vi "Turn To X -no loop.vi"(3 "STOP?":bool, 4 "Dest":u16, 5 "Start":u16, 6 "error in":errorcluster, 7 "FPGA VI Reference in":refnum<k20>) -> (0 "error out":errorcluster, 1 "FPGA VI Reference Out":refnum<k20>, 2 "x-y":i16)   [LabVIEW 2014]
uses:
  <vilib>/Utility/error.llb/Error Cluster From Error Code.vi
  <vilib>/rvi/errors/niLvFpgaAdjustHostInterfaceError.vi
  <vilib>/rvi/interface/nirviReadWriteControl/nirviReadWriteControl.xnode
  NiFpgaLv.dll
  <vilib>/rvi/interface/Simulation/niFpgaSimulationCallBeginRW.vi
panel:
  out "16bit integer":i16
  in  "Friction":dbl=1.0
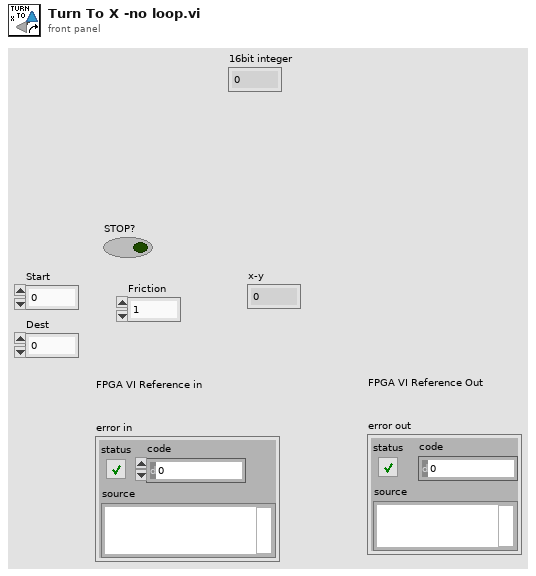
[diagram p1: front panel]
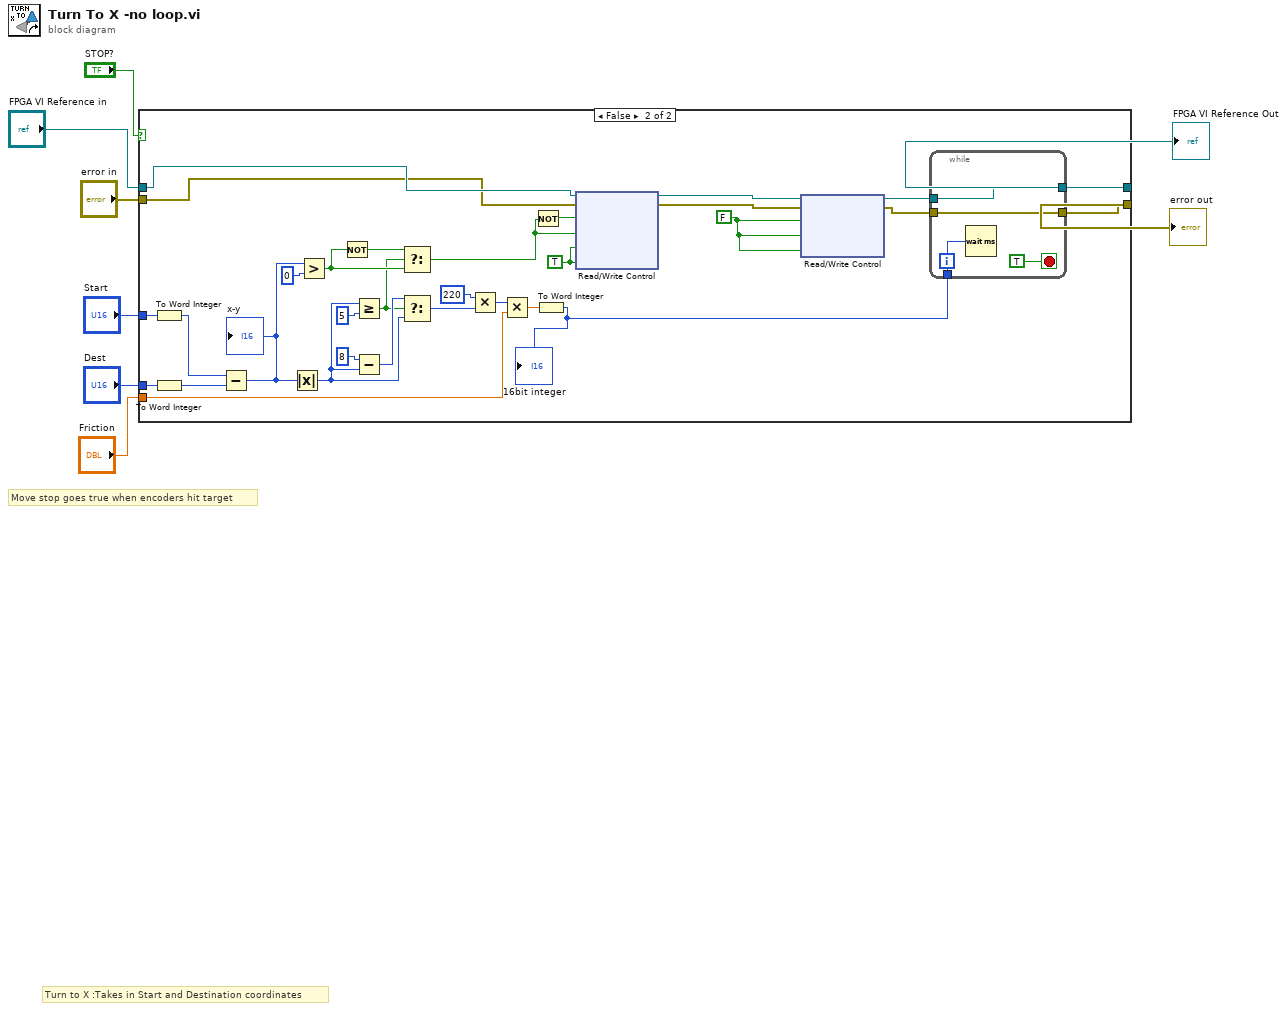
[diagram p0: block diagram]
diagram:
  # "Move stop goes true when encoders hit target"
  # "Turn to X :Takes in Start and Destination coordinates"
  n1 = case shown="False" "STOP?" {
    tunnel: "Start" -> [_ w40]
    tunnel: "Dest" -> [_ w37]
    tunnel: "error in" -> [w9 w13]
    tunnel: "FPGA VI Reference in" -> [w10 w14]
    tunnel: [w10 w19] -> w5
    tunnel: [w9 w17] -> w4
    tunnel: "Friction" -> [_ w41]
    frame True {
    }
    frame False {
      w20 = FALSE ("Stop Left")
      w21 = TRUE ("Right Motor")
      n2 = To Word Integer(number=w40) -> (16bit integer=w39:i16)
      n3 = To Word Integer(number=w37) -> (16bit integer=w38:i16)
      n4 = Subtract(x=w39, y=w38) -> (x-y=w34:i16)
      "x-y" <- w34
      n5 = Absolute Value(x=w34) -> (abs(x)=w22:i16)
      n6 = Greater?(x=w34, y=i16 0) -> (0:w25:bool)
      n7 = Not(x=w25) -> (.not. x?=w26:bool)
      n8 = Greater Or Equal?(x=w22, y=i16 5 ("x")) -> (x >= y?=w24:bool)
      n9 = Subtract(x=i16 8, y=w22) -> (x-y=w29:i16)
      n10 = Select(t=w26, s=w24, f=w25) -> (s? t:f=w11:bool)
      n11 = Select(t=w29, s=w24, f=w22) -> (s? t:f=w27:i16)
      n12 = Multiply(x=220 ("y"), y=w27) -> (x*y=w33:i32)
      n13 = Multiply(x=w33, y=w41) -> (x*y=w35:dbl)
      n14 = Not(x=w11) -> (.not. x?=w12:bool)
      n15 = To Word Integer(number=w35) -> (16bit integer=w15:i16)
      "16bit integer" <- w15
      n16 = xnode "Read/Write Control"("FPGA VI Reference In"=w14, "error in"=w13, "Left Motor"=w12, "Right Motor"=w11, "Stop Left"=w21, "Stop Right"=w21) -> ("FPGA VI Reference Out"=w32:refnum<k20>, "error out"=w31:errorcluster)
      n17 = xnode "Read/Write Control"("FPGA VI Reference In"=w32, "error in"=w31, "Stop Left"=w20, "Stop Right"=w20, "Stop motors"=w20) -> ("FPGA VI Reference Out"=w18:refnum<k20>, "error out"=w16:errorcluster)
      n18 = while {
        tunnel: [w45] -> w19
        tunnel: w18 -> [w45]
        tunnel: [w44] -> w17
        tunnel: w16 -> [w44]
        tunnel: w15 -> [w42]
        stop <- TRUE stop-if-true
        n19 = Wait (ms)(milliseconds to wait=w42) -> ()  [unwired: 1 out]
      }
    }
  }
  "FPGA VI Reference Out" <- w5
  "error out" <- w4
